vi "Sub_plotter.vi"(10 "Experiment":T3) -> (3 "Plotables":T1)   [LabVIEW 2021]
panel:
  out "Plotables":T2
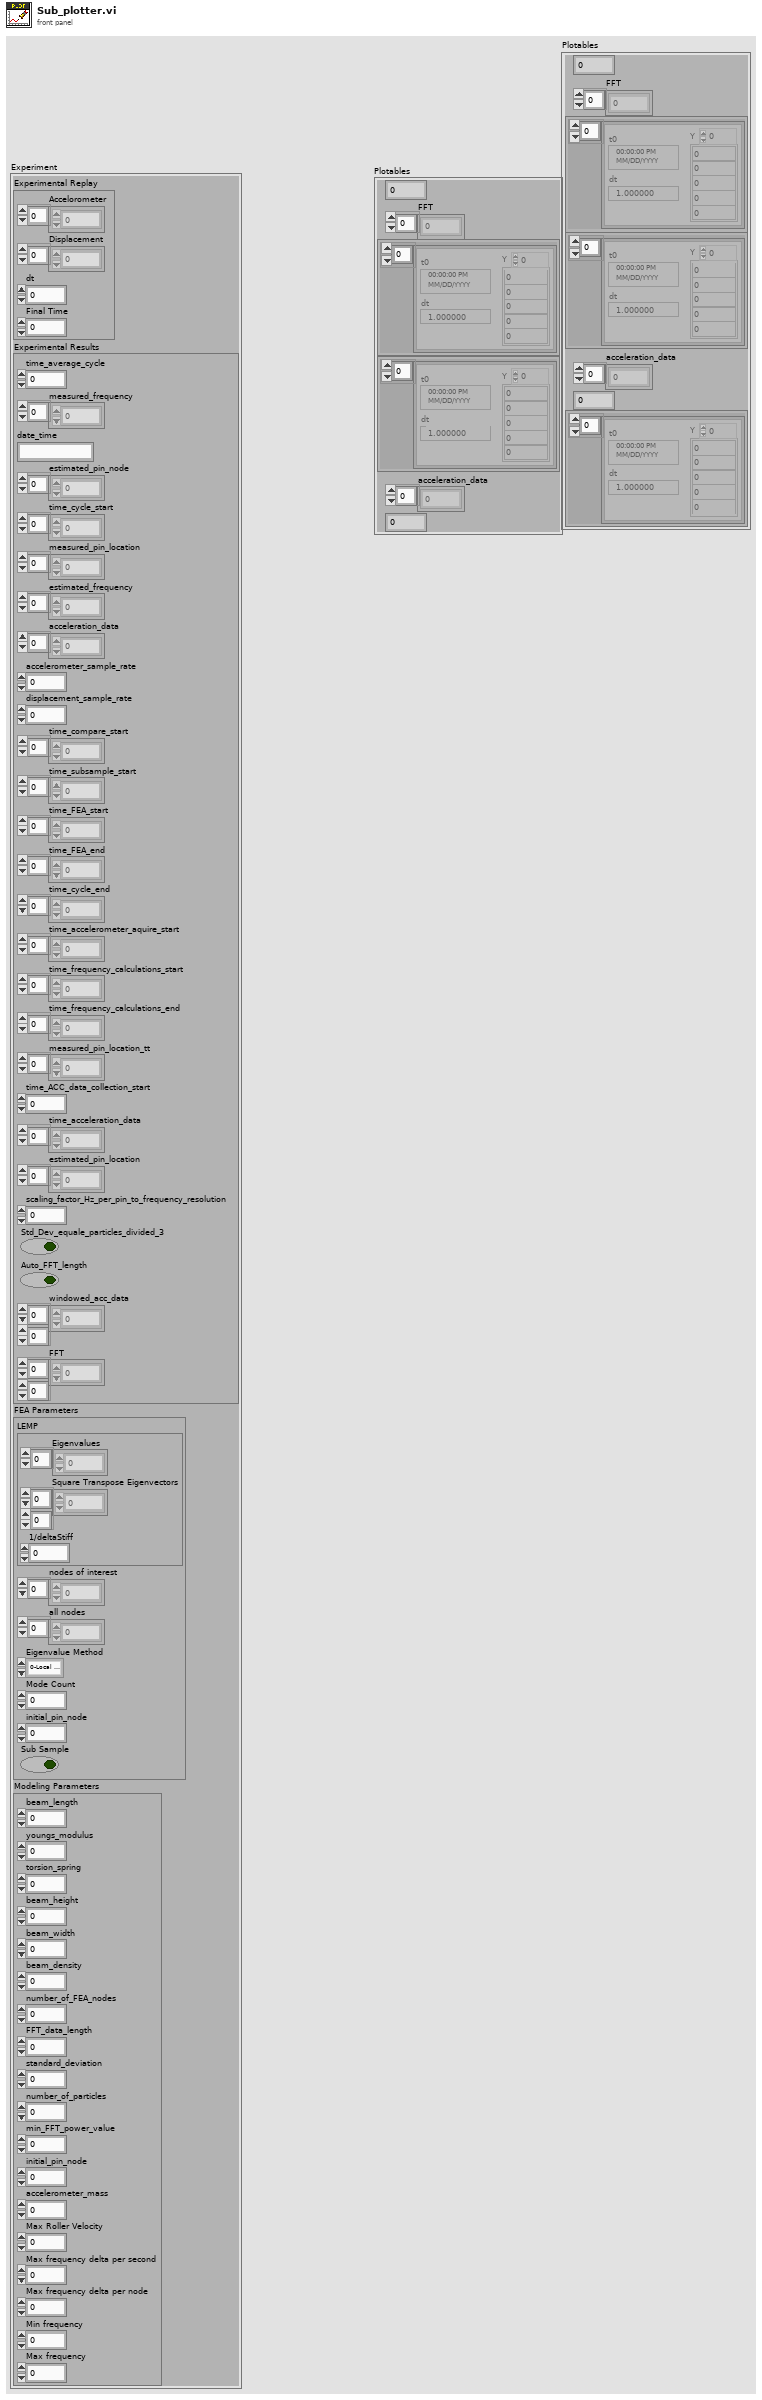
[diagram p1: front panel]
types:
  T1 = cluster{dbl, "FFT":dbl[], "Dynamic Data":dynamicdata, "Dynamic Data":dynamicdata, "acceleration_data":dbl[], dbl, "Dynamic Data":dynamicdata}
  T2 = cluster{dbl, "FFT":dbl[], "Dynamic Data":dynamicdata, "Dynamic Data":dynamicdata, "acceleration_data":dbl[], dbl}
  T3 = cluster{"Experimental Replay":cluster{"Accelorometer":dbl[], "Displacement":dbl[], "dt":dbl, "Final Time":dbl}, "Experimental Results":cluster{"time_average_cycle":dbl, "measured_frequency":dbl[], "date_time":string, "estimated_pin_node":i32[], "time_cycle_start":dbl[], "measured_pin_location":dbl[], "estimated_frequency":dbl[], "acceleration_data":dbl[], "accelerometer_sample_rate":dbl, "displacement_sample_rate":dbl, "time_compare_start":dbl[], "time_subsample_start":dbl[], "time_FEA_start":dbl[], "time_FEA_end":dbl[], "time_cycle_end":dbl[], "time_accelerometer_aquire_start":dbl[], "time_frequency_calculations_start":dbl[], "time_frequency_calculations_end":dbl[], "measured_pin_location_tt":dbl[], "time_ACC_data_collection_start":dbl, "time_acceleration_data":dbl[], "estimated_pin_location":dbl[], "scaling_factor_Hz_per_pin_to_frequency_resolution":dbl, "Std_Dev_equale_particles_divided_3":bool, "Auto_FFT_length":bool, "windowed_acc_data":dbl[][], "FFT":dbl[][]}, "FEA Parameters":cluster{"LEMP":cluster{"Eigenvalues":dbl[], "Square Transpose Eigenvectors":dbl[][], "1/deltaStiff":dbl}, "nodes of interest":i32[], "all nodes":i32[], "Eigenvalue Method":enum16{"0-Local Eigen Modification Procedure", "1-LabVIEW generalized eigenvalues", "2-LabVIEW M^-1K eigenvalues", "3-LabVIEW Cholesky Factorization", "4-Cholesky Factorization CPU SGL", "5-Cholesky Factorization CPU FXP", "6-Cholesky Factorization FPGA SGL", "7-Cholesky Factorization FPGA SGL SCL"}, "Mode Count":i32, "initial_pin_node":i32, "Sub Sample":bool}, "Modeling Parameters":cluster{"beam_length":dbl, "youngs_modulus":dbl, "torsion_spring":dbl, "beam_height":dbl, "beam_width":dbl, "beam_density":dbl, "number_of_FEA_nodes":i32, "FFT_data_length":i32, "standard_deviation":dbl, "number_of_particles":i32, "min_FFT_power_value":dbl, "initial_pin_node":i32, "accelerometer_mass":dbl, "Max Roller Velocity":dbl, "Max frequency delta per second":dbl, "Max frequency delta per node":dbl, "Min frequency":dbl, "Max frequency":dbl}}
  T4 = cluster{dbl, "FFT":dbl[], dynamicdata, dynamicdata, "acceleration_data":dbl[], dbl, dynamicdata}
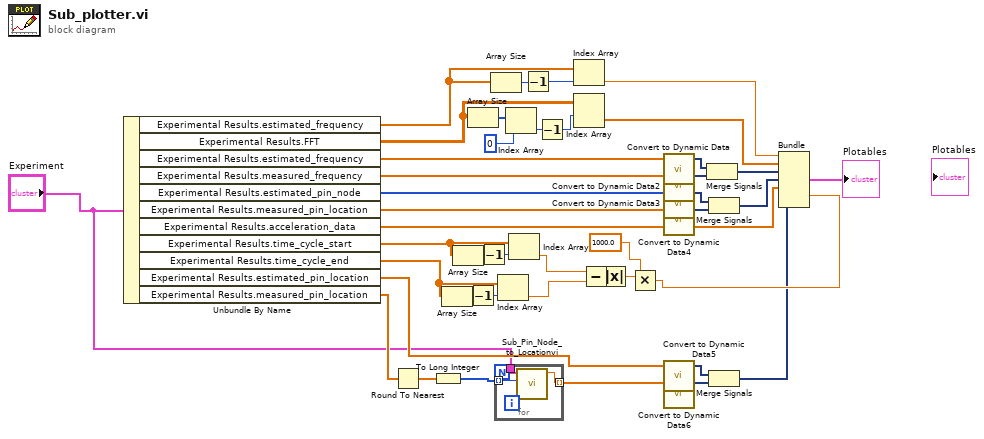
[diagram p0: block diagram]
diagram:
  n1 = Unbundle By Name("Experiment") -> ("Experimental Results.estimated_frequency"=w35:dbl[], "Experimental Results.FFT"=w39:dbl[][], "Experimental Results.estimated_frequency"=w41:dbl[], "Experimental Results.measured_frequency"=w40:dbl[], "Experimental Results.estimated_pin_node"=w42:i32[], "Experimental Results.measured_pin_location"=w43:dbl[], "Experimental Results.acceleration_data"=w13:dbl[], "Experimental Results.time_cycle_start"=w26:dbl[], "Experimental Results.time_cycle_end"=w21:dbl[], "Experimental Results.estimated_pin_location"=w5:dbl[], "Experimental Results.measured_pin_location"=w10:dbl[])
  n2 = Round To Nearest(number=w10) -> (nearest integer value=w9:dbl[])
  n3 = To Long Integer(number=w9) -> (32bit integer=w8:i32[])
  n4 = Array Size(array=w21) -> (size(s)=w23:i32)
  n5 = Array Size(array=w26) -> (size(s)=w25:i32)
  n6 = Array Size(array=w39) -> (size(s)=w38:i32[])
  n7 = Decrement(x=w23) -> (x-1=w22:i32)
  n8 = Decrement(x=w25) -> (x-1=w24:i32)
  n9 = Array Size(array=w35) -> (size(s)=w34:i32)
  n10 = for {
    tunnel: w8 -> [w46] mode=indexing
    tunnel: [w45] -> w4 mode=indexing
    tunnel: "Experiment" -> [w44]
    n11 = call "Sub_Pin_Node_to_Locationvi.vi"("Node"=w46, "Experiment in"=w44) -> ("Pin location"=w45:dbl)  [unwired: 9 in]
  }
  n12 = Index Array(array=w21, index=w22) -> (element=w20:dbl)
  n13 = Index Array(array=w38, index=0) -> (element=w36:i32)
  n14 = Index Array(array=w26, index=w24) -> (element=w19:dbl)
  n15 = Decrement(x=w34) -> (x-1=w33:i32)
  n16 = Decrement(x=w36) -> (x-1=w14:i32)
  n17 = Index Array(array=w35, index=w33) -> (element=w16:dbl)
  n18 = Index Array(array=w39, index (row)=w14) -> (element=w15:dbl[])  [unwired: 1 in]
  n19 = Subtract(x=w19, y=w20) -> (x-y=w32:dbl)
  n20 = Absolute Value(x=w32) -> (abs(x)=w31:dbl)
  n21 = Multiply(x=w31, y=1000.0) -> (x*y=w12:dbl)
  n22 = call "Convert to Dynamic Data"("Array"=w41) -> ("Dynamic Data Type"=w30:dynamicdata)  [unwired: 3 in]
  n23 = call "Convert to Dynamic Data2"("Array"=w40) -> ("Dynamic Data Type"=w29:dynamicdata)  [unwired: 3 in]
  n24 = call "Convert to Dynamic Data3"("Array"=w42) -> ("Dynamic Data Type"=w28:dynamicdata)  [unwired: 3 in]
  n25 = call "Convert to Dynamic Data4"("Array"=w43) -> ("Dynamic Data Type"=w27:dynamicdata)  [unwired: 3 in]
  n26 = call "Convert to Dynamic Data5"("Array"=w5) -> ("Dynamic Data Type"=w7:dynamicdata)  [unwired: 3 in]
  n27 = call "Convert to Dynamic Data6"("Array"=w4) -> ("Dynamic Data Type"=w6:dynamicdata)  [unwired: 3 in]
  n28 = Merge Signals(w30, w29) -> (w18:dynamicdata)
  n29 = Merge Signals(w28, w27) -> (w17:dynamicdata)
  n30 = Merge Signals(w7, w6) -> (w2:dynamicdata)
  n31 = Bundle(w16, "FFT"=w15, w18, w17, "acceleration_data"=w13, w12, w2) -> (→"Plotables":T4)  [unwired: 1 in]
